vi "Set Generic Property.vi"(0 "SLSC Interface in":refnum<class "SLSC Interface.lvclass">, 1 "property type":T1, 5 "resources":string, 7 "property":refnum<k21>, 9 "property value":variant, 11 "error in (no error)":errorcluster) -> (4 "SLSC Interface out":refnum<class "SLSC Interface.lvclass">, 15 "error out":errorcluster)   [LabVIEW 2015, in "SLSC Interface.lvclass"]
uses:
  SLSC Interface.lvclass
  property type.ctl
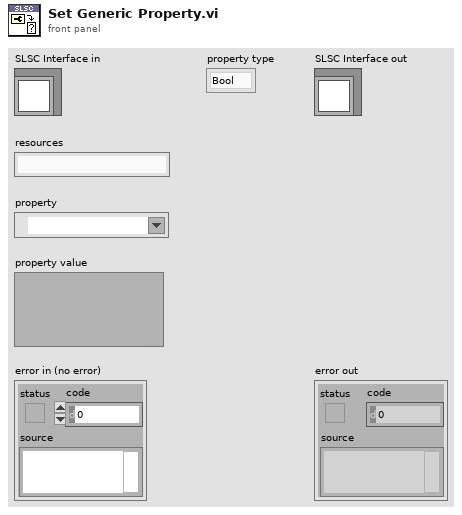
[diagram p1: front panel]
types:
  T1 = typedef "SLSC Interface.lvclass/property type.ctl" = enum16{"Bool", "DBL", "I32", "I64", "String", "U32", "U64", "1D Bool", "1D DBL", "1D I32", "1D I64", "1D String", "1D U32", "1D U64"}
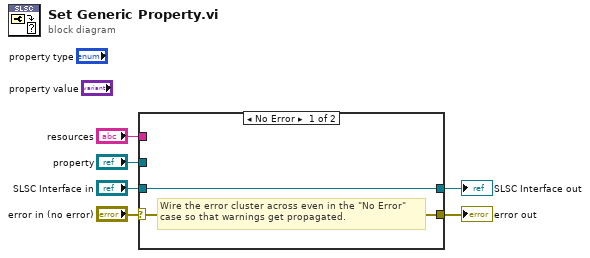
[diagram p0: block diagram]
diagram:
  n1 = case shown="No Error" "error in (no error)" {
    selector: "error in (no error)" -> [w7 w10]
    tunnel: [w7 w10] -> w5
    tunnel: [w8 w9] -> w3
    tunnel: "SLSC Interface in" -> [w8 w9]
    tunnel: "resources" -> [_ _]
    tunnel: "property" -> [_ _]
    frame No Error {
      # "Wire the error cluster across even in the \"No Error\"\ncase so that warnings get propagated."
    }
    frame Error {
    }
  }
  "error out" <- w5
  "SLSC Interface out" <- w3
